vi "1D Cluster to Color Table.vi"(9 "Show Cell Index? (T)":bool=TRUE, 10 "1D Board":T1[](array[typedef])=[{"Team"=0, "Occu."=enum."N", "Count"=0}, {"Team"=0, "Occu."=enum."N", "Count"=0}, {"Team"=1, "Occu."=enum."C", "Count"=1}, {"Team"=0, "Occu."=enum."N", "Count"=0}, {"Team"=1, "Occu."=enum."N", "Count"=1}, {"Team"=1, "Occu."=enum."C", "Count"=0}, {"Team"=1, "Occu."=enum."N", "Count"=1}, {"Team"=0, "Occu."=enum."N", "Count"=0}, {"Team"=0, "Occu."=enum."N", "Count"=0}, {"Team"=0, "Occu."=enum."N", "Count"=0}, {"Team"=0, "Occu."=enum."N", "Count"=0}, {"Team"=1, "Occu."=enum."K", "Count"=0}, {"Team"=1, "Occu."=enum."C", "Count"=2}, {"Team"=1, "Occu."=enum."C", "Count"=1}, {"Team"=0, "Occu."=enum."N", "Count"=0}, {"Team"=2, "Occu."=enum."C", "Count"=1}, {"Team"=0, "Occu."=enum."N", "Count"=0}, {"Team"=0, "Occu."=enum."N", "Count"=0}, {"Team"=0, "Occu."=enum."N", "Count"=0}, {"Team"=1, "Occu."=enum."C", "Count"=1}, {"Team"=0, "Occu."=enum."N", "Count"=0}, {"Team"=2, "Occu."=enum."C", "Count"=1}, {"Team"=2, "Occu."=enum."C", "Count"=1}, {"Team"=2, "Occu."=enum."C", "Count"=1}, {"Team"=2, "Occu."=enum."C", "Count"=1}, {"Team"=0, "Occu."=enum."N", "Count"=0}, {"Team"=0, "Occu."=enum."N", "Count"=0}, {"Team"=0, "Occu."=enum."N", "Count"=0}, {"Team"=2, "Occu."=enum."C", "Count"=1}, {"Team"=0, "Occu."=enum."N", "Count"=0}, {"Team"=1, "Occu."=enum."C", "Count"=1}, {"Team"=0, "Occu."=enum."N", "Count"=0}, {"Team"=1, "Occu."=enum."C", "Count"=1}, {"Team"=0, "Occu."=enum."N", "Count"=0}, {"Team"=0, "Occu."=enum."N", "Count"=0}, {"Team"=2, "Occu."=enum."C", "Count"=1}, {"Team"=0, "Occu."=enum."N", "Count"=0}, {"Team"=0, "Occu."=enum."N", "Count"=0}, {"Team"=0, "Occu."=enum."N", "Count"=0}, {"Team"=0, "Occu."=enum."N", "Count"=0}, {"Team"=0, "Occu."=enum."N", "Count"=0}, {"Team"=1, "Occu."=enum."C", "Count"=1}, {"Team"=0, "Occu."=enum."N", "Count"=0}, {"Team"=0, "Occu."=enum."N", "Count"=0}, {"Team"=1, "Occu."=enum."C", "Count"=1}, {"Team"=1, "Occu."=enum."C", "Count"=1}, {"Team"=0, "Occu."=enum."N", "Count"=0}, {"Team"=0, "Occu."=enum."N", "Count"=0}, {"Team"=0, "Occu."=enum."N", "Count"=0}], 11 "Debug Board 2D String Ref":refnum<vi>) -> ()   [LabVIEW 2014, in "Dragon Tamers.lvlib"]
uses:
  Typedefs/Board Cell.ctl
  Typedefs/Cell Occupancy.ctl
  <vilib>/Utility/miscctls.llb/LVRowAndColumnTypeDef.ctl
  Dragon Tamers.lvlib
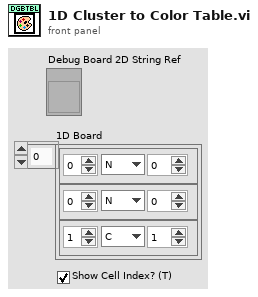
[diagram p1: front panel]
types:
  T1 = typedef "Dragon Tamers.lvlib/Board Cell.ctl" = cluster{"Team":i32, "Occu.":T2, "Count":i32}
  T2 = typedef "Dragon Tamers.lvlib/Cell Occupancy.ctl" = enum16{"N", "C", "K"}
  T3 = typedef "Dragon Tamers.lvlib/Debug Board 2D String.ctl" = string[][]
  T4 = typedef "Debug Board 2D String.ctl" = string[][]
  T5 = typedef "LVRowAndColumnTypeDef.ctl" = cluster{"Row":i32, "Column":i32}
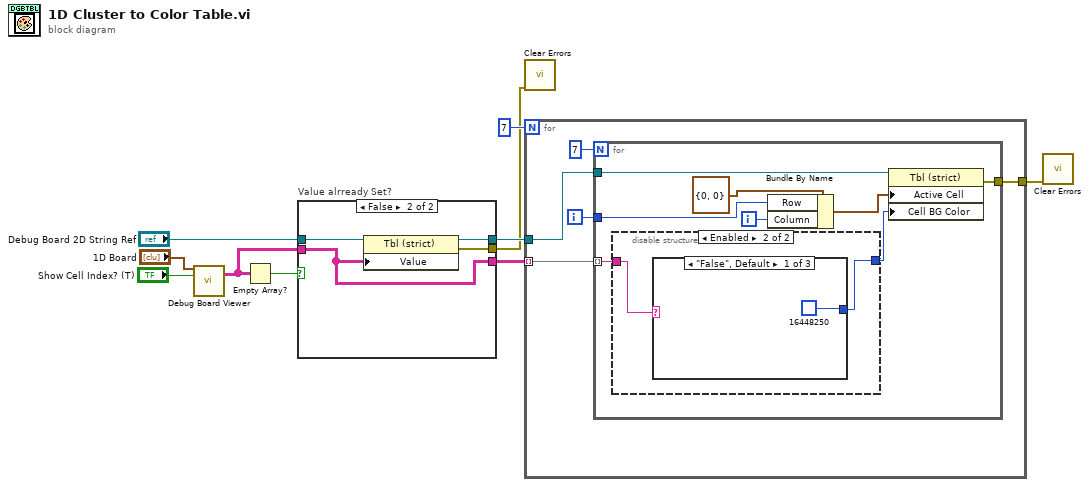
[diagram p0: block diagram]
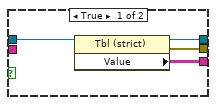
[diagram p2: hidden frame]
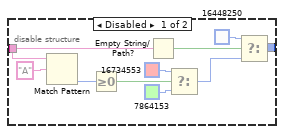
[diagram p3: hidden frame]
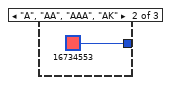
[diagram p4: hidden frame]
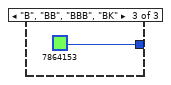
[diagram p5: hidden frame]
diagram:
  n1 = call "Debug Board Viewer.vi"("1D Board"="1D Board", "Show Cell Index?"="Show Cell Index? (T)") -> ("Debug Board 2D String"=w3:T3)  [unwired: 12 in, 1 out]
  n2 = Empty Array?(array=w3) -> (empty?=w8:bool)
  n3 = case "Value alrready Set?" shown="False" w8 {
    tunnel: w3 -> [_ w17]
    tunnel: "Debug Board 2D String Ref" -> [w14 w18]
    tunnel: [w13 w17] -> w4
    tunnel: [w12 w16] -> w6
    tunnel: [w11 w15] -> w5
    frame True {
      n4 = property class="Tbl (strict)"(reference=w14) -> (reference out=w12:refnum<vi>, error out=w11:errorcluster, "Value"=w13:T4)  [unwired: 1 in]
    }
    frame False {
      n5 = property class="Tbl (strict)"(reference=w18, "Value"=w17) -> (reference out=w16:refnum<vi>, error out=w15:errorcluster)  [unwired: 1 in]
    }
  }
  n6 = call <vilib>:"Clear Errors.vi"("error in (no error)"=w5) -> ()  [unwired: 5 in, 2 out]
  n7 = for {
    N: 7 -> [_]
    tunnel: w6 -> [w23]
    tunnel: w4 -> [w20] mode=indexing
    tunnel: [w19] -> w9
    i -> [w21]
    n8 = for {
      N: 7 -> [_]
      tunnel: w23 -> [w31]
      tunnel: w21 -> [w29]
      tunnel: w20 -> [w26] mode=indexing
      tunnel: [w24] -> w19
      i -> [w28]
      n9 = disable-structure shown="Enabled" {
        disable-tunnel: w26 -> [w41 w43]
        disable-tunnel: [w33 w42] -> w25
        frame Disabled {
          n10 = Match Pattern(string=w41, regular expression="A") -> (offset past match=w39:i32)  [unwired: 1 in, 3 out]
          n11 = Greater Or Equal To 0?(x=w39) -> (x >= 0?=w38:bool)
          n12 = Empty String/Path?(string/path=w41) -> (empty?=w35:bool)
          n13 = Select(t=u32 16734553 ("Color Box"), s=w38, f=u32 7864153 ("Color Box")) -> (s? t:f=w34:u32)
          n14 = Select(t=u32 16448250 ("Color Box"), s=w35, f=w34) -> (s? t:f=w33:u32)
        }
        frame Enabled {
          n15 = case shown="\"False\", Default" w43 {
            tunnel: [u32 16448250 ("Color Box") u32 16734553 ("Color Box") u32 7864153 ("Color Box")] -> w42
            frame "False", Default {
            }
            frame "A", "AA", "AAA", "AK" {
            }
            frame "B", "BB", "BBB", "BK" {
            }
          }
        }
      }
      n16 = Bundle By Name(cluster=T5 {"Row"=0, "Column"=0} ("Active Cell:Active Cell"), "Row"=w29, "Column"=w28) -> (w27:T5)
      n17 = property class="Tbl (strict)"(reference=w31, "Active Cell"=w27, "Cell BG Color"=w25) -> (error out=w24:errorcluster)  [unwired: 1 in, 1 out]
    }
  }
  n18 = call <vilib>:"Clear Errors.vi"("error in (no error)"=w9) -> ()  [unwired: 5 in, 2 out]
